vi "Set stack field.vi"(7 "Is Module?":bool, 8 "error in (no error)":errorcluster, 9 "Value in":string, 10 "Field":string, 11 "Stack in":refnum<class "Stack.lvclass">) -> (0 "error out":errorcluster, 3 "Stack out":refnum<class "Stack.lvclass">)   [LabVIEW 2021, in "Stack.lvclass"]
uses:
  Stack.lvclass
  Stack.lvclass/Stack.ctl
panel:
  out "String":string
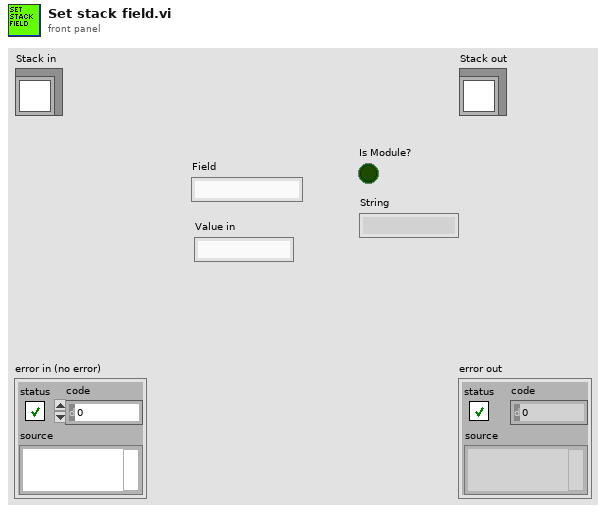
[diagram p1: front panel]
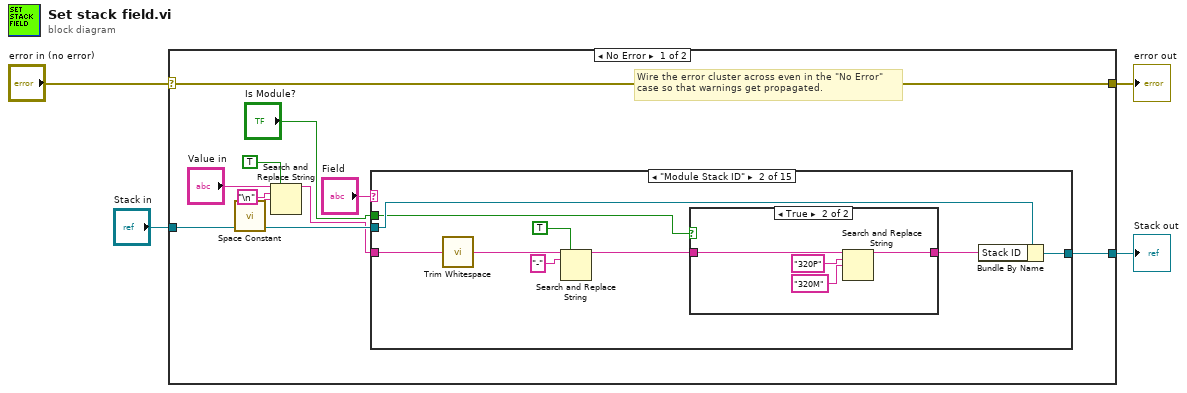
[diagram p0: block diagram]
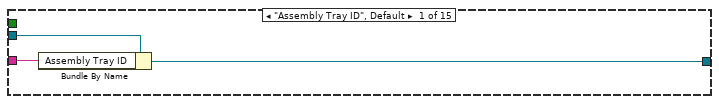
[diagram p2: hidden frame]
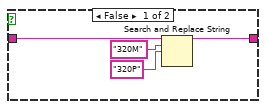
[diagram p3: hidden frame]
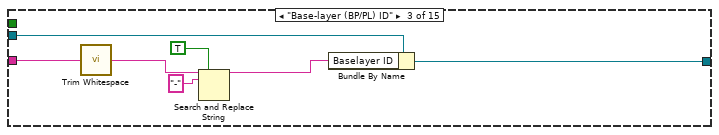
[diagram p4: hidden frame]
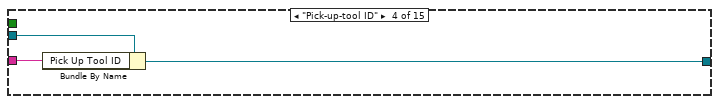
[diagram p5: hidden frame]
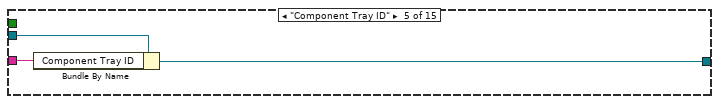
[diagram p6: hidden frame]
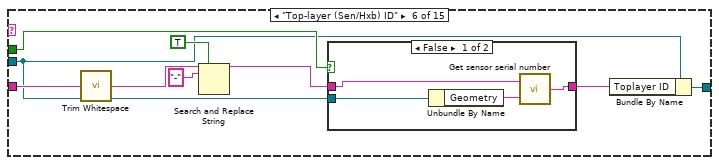
[diagram p7: hidden frame]
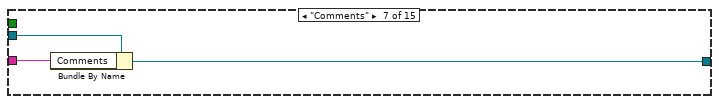
[diagram p9: hidden frame]
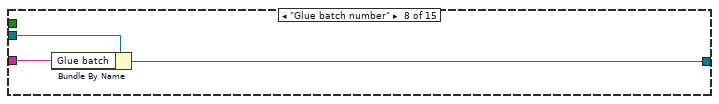
[diagram p10: hidden frame]
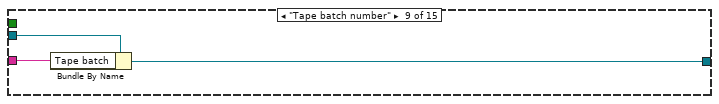
[diagram p11: hidden frame]
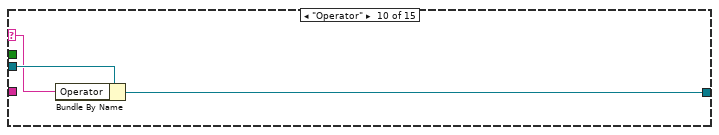
[diagram p12: hidden frame]
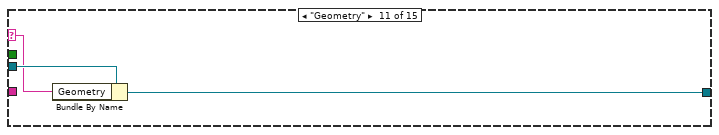
[diagram p13: hidden frame]
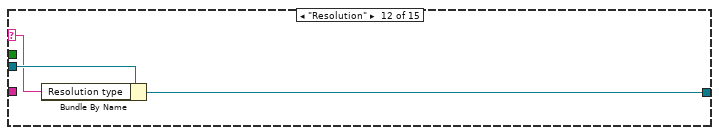
[diagram p14: hidden frame]
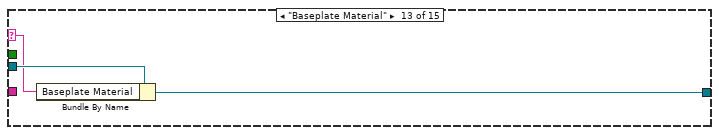
[diagram p15: hidden frame]
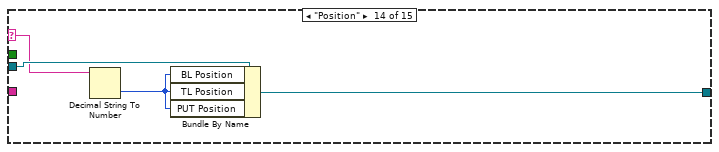
[diagram p16: hidden frame]
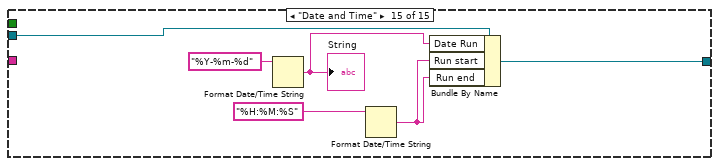
[diagram p17: hidden frame]
diagram:
  n1 = case shown="No Error" "error in (no error)" {
    selector: "error in (no error)" -> [w14 w94]
    tunnel: [w14 w94] -> w3
    tunnel: [w12 w93] -> w1
    tunnel: "Stack in" -> [w13 w93]
    frame No Error {
      # "Wire the error cluster across even in the \"No Error\"\ncase so that warnings get propagated."
      n2 = call <vilib>:"Space Constant.vi"() -> ("String"=w7:string)
      n3 = Search and Replace String(replace all?=TRUE ("replace all? (F)"), input string="Value in", search string="\n", replace string=w7) -> (result string=w5:string)  [unwired: 4 in, 3 out]
      n4 = case shown="\"Module Stack ID\"" "Field" {
        selector: "Field" -> [_ _ _ _ _ _ _ _ _ w71 w74 w77 w80 w84 _]
        tunnel: w13 -> [w17 w26 w41 w44 w47 w48 w64 w67 w70 w73 w76 w79 w82 w86 w92]
        tunnel: [w16 w25 w40 w43 w46 w56 w63 w66 w69 w72 w75 w78 w81 w85 w91] -> w12
        tunnel: w5 -> [w15 w24 w36 w42 w45 w52 w62 w65 w68 _ _ _ _ _ _]
        tunnel: "Is Module?" -> [_ w21 _ _ _ w51 _ _ _ _ _ _ _ _ _]
        frame "Assembly Tray ID", Default {
          n5 = Bundle By Name(cluster=w17, "Assembly Tray ID"=w15) -> (w16:refnum<class "Stack.lvclass">)
        }
        frame "Module Stack ID" {
          n6 = call <vilib>:"Trim Whitespace.vi"("string"=w24) -> ("trimmed string"=w18:string)  [unwired: 1 in]
          n7 = Search and Replace String(replace all?=TRUE ("replace all? (F)"), input string=w18, search string="-") -> (result string=w20:string)  [unwired: 5 in, 3 out]
          n8 = case shown="True" w21 {
            tunnel: w20 -> [w30 w32]
            tunnel: [w29 w31] -> w19
            frame False {
              n9 = Search and Replace String(input string=w30, search string="320M", replace string="320P" ("replace string (\"\")")) -> (result string=w29:string)  [unwired: 5 in, 3 out]
            }
            frame True {
              n10 = Search and Replace String(input string=w32, search string="320P", replace string="320M" ("replace string (\"\")")) -> (result string=w31:string)  [unwired: 5 in, 3 out]
            }
          }
          n11 = Bundle By Name(cluster=w26, "Stack ID"=w19) -> (w25:refnum<class "Stack.lvclass">)
        }
        frame "Base-layer (BP/PL) ID" {
          n12 = call <vilib>:"Trim Whitespace.vi"("string"=w36) -> ("trimmed string"=w37:string)  [unwired: 1 in]
          n13 = Search and Replace String(replace all?=TRUE ("replace all? (F)"), input string=w37, search string="-") -> (result string=w35:string)  [unwired: 5 in, 3 out]
          n14 = Bundle By Name(cluster=w41, "Baselayer ID"=w35) -> (w40:refnum<class "Stack.lvclass">)
        }
        frame "Pick-up-tool ID" {
          n15 = Bundle By Name(cluster=w44, "Pick Up Tool ID"=w42) -> (w43:refnum<class "Stack.lvclass">)
        }
        frame "Component Tray ID" {
          n16 = Bundle By Name(cluster=w47, "Component Tray ID"=w45) -> (w46:refnum<class "Stack.lvclass">)
        }
        frame "Top-layer (Sen/Hxb) ID" {
          n17 = call <vilib>:"Trim Whitespace.vi"("string"=w52) -> ("trimmed string"=w53:string)  [unwired: 1 in]
          n18 = Search and Replace String(replace all?=TRUE ("replace all? (F)"), input string=w53, search string="-") -> (result string=w49:string)  [unwired: 5 in, 3 out]
          n19 = case shown="False" w51 {
            tunnel: [w60 w61] -> w50
            tunnel: w49 -> [w59 w61]
            tunnel: w48 -> [w58 _]
            frame False {
              n20 = Unbundle By Name(w58) -> ("Geometry"=w57:string)
              n21 = call "Get sensor serial number.vi"("Geometry"=w57, "Toplayer ID"=w59) -> ("Toplayer ID out"=w60:string)
            }
            frame True {
            }
          }
          n22 = Bundle By Name(cluster=w48, "Toplayer ID"=w50) -> (w56:refnum<class "Stack.lvclass">)
        }
        frame "Comments" {
          n23 = Bundle By Name(cluster=w64, "Comments"=w62) -> (w63:refnum<class "Stack.lvclass">)
        }
        frame "Glue batch number" {
          n24 = Bundle By Name(cluster=w67, "Glue batch"=w65) -> (w66:refnum<class "Stack.lvclass">)
        }
        frame "Tape batch number" {
          n25 = Bundle By Name(cluster=w70, "Tape batch"=w68) -> (w69:refnum<class "Stack.lvclass">)
        }
        frame "Operator" {
          n26 = Bundle By Name(cluster=w73, "Operator"=w71) -> (w72:refnum<class "Stack.lvclass">)
        }
        frame "Geometry" {
          n27 = Bundle By Name(cluster=w76, "Geometry"=w74) -> (w75:refnum<class "Stack.lvclass">)
        }
        frame "Resolution" {
          n28 = Bundle By Name(cluster=w79, "Resolution type"=w77) -> (w78:refnum<class "Stack.lvclass">)
        }
        frame "Baseplate Material" {
          n29 = Bundle By Name(cluster=w82, "Baseplate Material"=w80) -> (w81:refnum<class "Stack.lvclass">)
        }
        frame "Position" {
          n30 = Decimal String To Number(string=w84) -> (number=w83:i32)  [unwired: 2 in, 1 out]
          n31 = Bundle By Name(cluster=w86, "BL Position"=w83, "TL Position"=w83, "PUT Position"=w83) -> (w85:refnum<class "Stack.lvclass">)
        }
        frame "Date and Time" {
          n32 = Format Date/Time String(time format string (%c)="%Y-%m-%d") -> (date/time string=w87:string)  [unwired: 2 in]
          "String" <- w87
          n33 = Format Date/Time String(time format string (%c)="%H:%M:%S") -> (date/time string=w89:string)  [unwired: 2 in]
          n34 = Bundle By Name(cluster=w92, "Date Run"=w87, "Run start"=w89, "Run end"=w89) -> (w91:refnum<class "Stack.lvclass">)
        }
      }
    }
    frame Error {
    }
  }
  "error out" <- w3
  "Stack out" <- w1
